vi "Agilent 2000 3000 X-Series Clock Recovery Jitter Measurement.vi"() -> ()   [LabVIEW 2015]
doc: "This example shows how to configure a 6000-X series oscilloscope to take a clock TIE jitter measurement.\n\n<b>Note:</b>\nThis example is specific to the 6000-X Series oscilloscopes. These features are not available on other models."
uses:
  Agilent 2000 3000 X-Series.lvlib
  Public/Data/Read Jitter Measurement (Clock TIE).vi
  Public/Configure/Math/Configure Clock Recovery (Explicit).vi
panel:
  in  "Edges (0: Rising)":u16(ring) items=["Rising", "Falling", "Either"]
  in  "Multiplier (1)":i32=1
  in  "Source (1: Channel 1)":u16(ring)=1 items=["Channel 1"=1, "Channel 2"=2, "Channel 3"=3, "Channel 4"=4]
  in  "Enable Clock Recovery (T: Enable)":bool=TRUE
  out "Clock TIE":dbl
  in  "Time Scale (0.0001 Sec/div)":dbl=0.0001
  in  "Waveform Generator Number (1: Waveform Generator 1)":i32(ring)=2 items=["Waveform Generator 1"=1, "Waveform Generator 2"=2]
  in  "Slope Clock TIE (0: Rising)":u16(ring) items=["Rising", "Falling", "Both"]
  in  "Units Clock TIE (0: Seconds)":u16(ring) items=["Seconds", "Unit Interval"]
  in  "Source Clock TIE (0: Channel 1)":u16(ring) items=["Channel 1", "Channel 2", "Channel 3", "Channel 4", "Math 1", "Math 2", "Math 3", "Math 4", "Reference Waveform 1", "Reference Waveform 2", "Reference Waveform 3", "Reference Waveform 4"]
  in  "Enable Output (T: Enable)":bool=TRUE
  in  "Frequency (1000 Hz)":dbl=10000000.0
  in  "Function Type (0: Sine)":i32(ring)=1 items=["Sine", "Square", "Ramp", "Pulse", "Noise", "DC", "Sine Cardinal", "Exponential Rise", "Exponential Fall", "Cardiac", "Gaussian Pulse", "Arbitrary"]
  in  "Math Function Index (1: Math Function 1)":i32(ring)=1 items=["Math Function 1"=1, "Math Function 2"=2, "Math Function 3"=3, "Math Function 4"=4]
  in  "Enable Display (T: Enable)":bool=TRUE
  in  "Math Operation (0: Add)":i32(ring)=26 items=["Add", "Subtract", "Multiply", "Integrate", "Diff", "FFT", "SQRT", "Magnify", "Absolute", "Square", "LN", "LOG", "EXP", "TEN", "Lowpass", "Highpass", "Divide", "Linear", "Trend", "Btiming", "Bstate", "Envelope", "Smoothing", "Max Hold", "Min Hold", "Average", "Clock Recovery"]
  in  "VISA resource name":refnum<visa-resource-name>
  # "(c) 2011-2023 National Instruments.  ALL RIGHTS RESERVED."
  # "Wave Generator Configuration"
  # "Clock Recovery Configuration"
  # "Clock TIE Measurement Configuration"
  # "Scale Configuration"
  # "Measured Clock TIE Value"
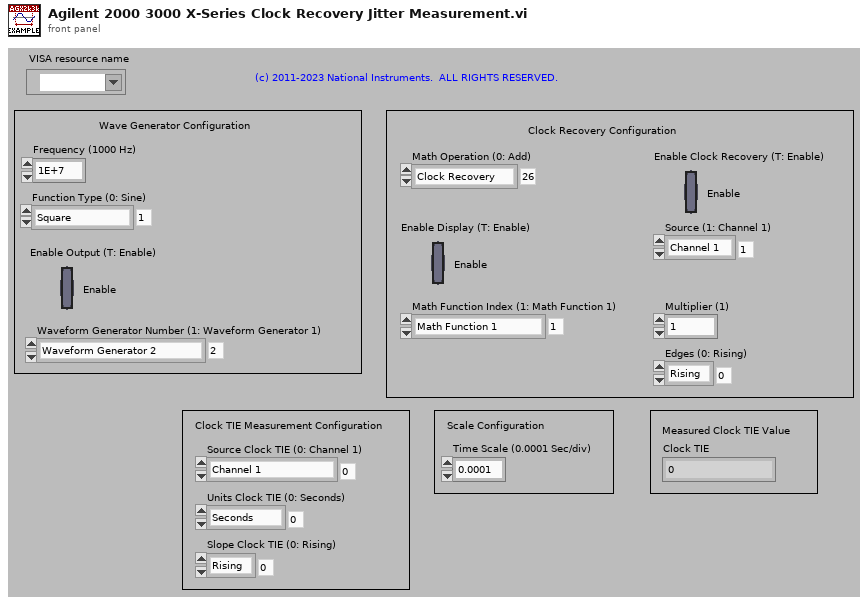
[diagram p1: front panel]
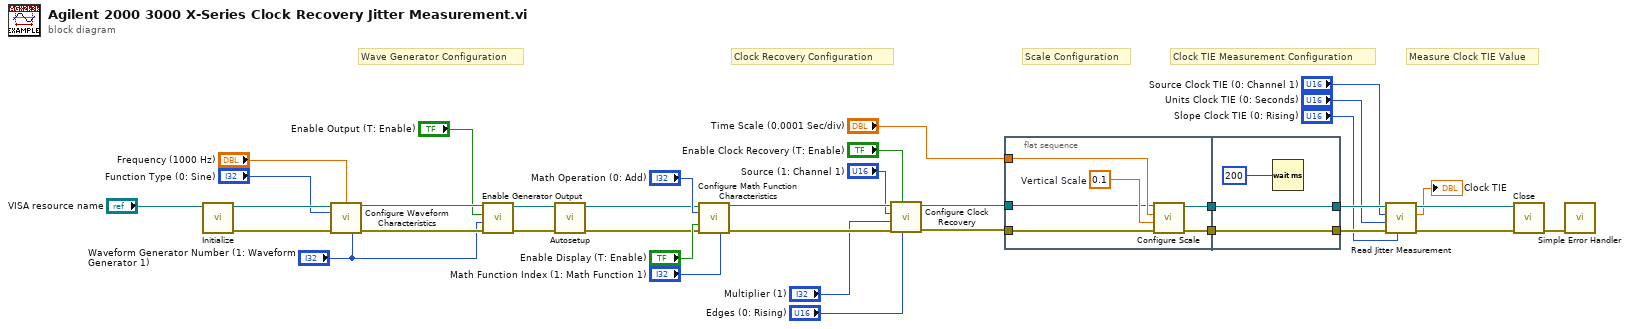
[diagram p0: block diagram]
diagram:
  # "Measure Clock TIE Value"
  # "Scale Configuration"
  # "Clock TIE Measurement Configuration"
  # "Clock Recovery Configuration"
  # "Wave Generator Configuration"
  n1 = call "Initialize.vi"("VISA resource name"="VISA resource name") -> ("error out"=w31:errorcluster, "VISA resource name out"=w32:refnum<visa-resource-name>)  [unwired: 9 in]
  n2 = call "Configure Waveform Characteristics.vi"("VISA resource name"=w32, "Frequency (1000 Hz)"="Frequency (1000 Hz)", "Function Type (0: Sine)"="Function Type (0: Sine)", "error in (no error)"=w31, "Waveform Generator Number (1: Waveform Generator 1)"="Waveform Generator Number (1: Waveform Generator 1)") -> ("VISA resource name out"=w30:refnum<visa-resource-name>, "error out"=w29:errorcluster)  [unwired: 9 in]
  n3 = call "Enable Generator Output.vi"("error in (no error)"=w29, "Waveform Generator Number (1: Waveform Generator 1)"="Waveform Generator Number (1: Waveform Generator 1)", "Enable Output (F: Disable)"="Enable Output (T: Enable)", "VISA resource name"=w30) -> ("error out"=w27:errorcluster, "VISA resource name out"=w28:refnum<visa-resource-name>)  [unwired: 6 in]
  n4 = call "Autosetup.vi"("error in (no error)"=w27, "VISA resource name"=w28) -> ("error out"=w25:errorcluster, "VISA resource name out"=w26:refnum<visa-resource-name>)  [unwired: 8 in]
  n5 = call "Configure Math Function Characteristics.vi"("VISA resource name"=w26, "Math Operation (0: Add)"="Math Operation (0: Add)", "Enable Display (T: Enable)"="Enable Display (T: Enable)", "error in (no error)"=w25, "Math Function Index (1: Math Function 1)"="Math Function Index (1: Math Function 1)") -> ("VISA resource name out"=w8:refnum<visa-resource-name>, "error out"=w6:errorcluster)  [unwired: 9 in]
  n6 = call-poly "Configure Clock Recovery.vi"("Edges (0: Rising)"="Edges (0: Rising)", "Enable Clock Recovery (T: Enable)"="Enable Clock Recovery (T: Enable)", "error in (no error)"=w6, "Multiplier (1)"="Multiplier (1)", "Source (1: Channel 1)"="Source (1: Channel 1)", "VISA resource name"=w8) -> ("error out"=w5:errorcluster, "VISA resource name out"=w7:refnum<visa-resource-name>)  [unwired: 4 in]
  n7 = flat-sequence {
    tunnel: w5 -> [w42]
    tunnel: [w41] -> w19
    tunnel: [w40] -> w18
    tunnel: "Time Scale (0.0001 Sec/div)" -> [w38]
    tunnel: w7 -> [w37]
    tunnel: [w44] -> w16
    tunnel: [w45] -> w17
    tunnel: w19 -> [w45]
    tunnel: w18 -> [w44]
    frame #0 {
      w39 = 0.1  # Vertical Scale
      n8 = call "Configure Scale.vi"("error in (no error)"=w42, "Vertical Scale (5 V/div)"=w39, "Time Scale (0.0001 Sec/div)"=w38, "VISA resource name"=w37) -> ("error out"=w40:errorcluster, "VISA resource name out"=w41:refnum<visa-resource-name>)  [unwired: 6 in]
    }
    frame #1 {
      n9 = Wait (ms)(milliseconds to wait=u32 200) -> ()  [unwired: 1 out]
    }
  }
  n10 = call-poly "Read Jitter Measurement.vi"("Slope Clock TIE (0: Rising)"="Slope Clock TIE (0: Rising)", "error in (no error)"=w16, "Units Clock TIE (0: Seconds)"="Units Clock TIE (0: Seconds)", "Source Clock TIE (0: Channel 1)"="Source Clock TIE (0: Channel 1)", "VISA resource name"=w17) -> ("error out"=w11:errorcluster, "Clock TIE"=→"Clock TIE":dbl, "VISA resource name out"=w12:refnum<visa-resource-name>)  [unwired: 4 in]
  n11 = call "Close.vi"("error in (no error)"=w11, "VISA resource name"=w12) -> ("error out"=w20:errorcluster)  [unwired: 9 in]
  n12 = call <vilib>:"Simple Error Handler.vi"("error in (no error)"=w20) -> ()  [unwired: 4 in, 5 out]
